vi "Test_WriteValue_InvalidType_Error.vi"(8 "error in (no error)":errorcluster, 11 "TestFormattedStringBinding In":refnum<class "TestFormattedStringBinding.lvclass">) -> (0 "error out":errorcluster, 3 "TestFormattedStringBinding Out":refnum<class "TestFormattedStringBinding.lvclass">)   [LabVIEW 2017, in "TestFormattedStringBinding.lvclass"]
uses:
  TestFormattedStringBinding.lvclass
  Source/Concrete/FormattedStringBinding/FormattedStringBinding.lvclass/FormattedStringBinding.ctl
  Source/Concrete/FormattedStringBinding/FormattedStringBinding.lvclass
  C:/Git/composed-transport/Source/Concrete/TerminalValueBinding/TerminalValueBinding.lvclass
  C:/Git/composed-transport/Source/ITransport/ITransport.lvclass
  <vilib>/Utility/error.llb/Error Cluster From Error Code.vi
  Source/Concrete/TerminalValueBinding/Construct Terminal Value Binding.vi
  Source/ITransport/ITransport.lvclass
panel:
  in  "String":string
  out "Return Error":errorcluster
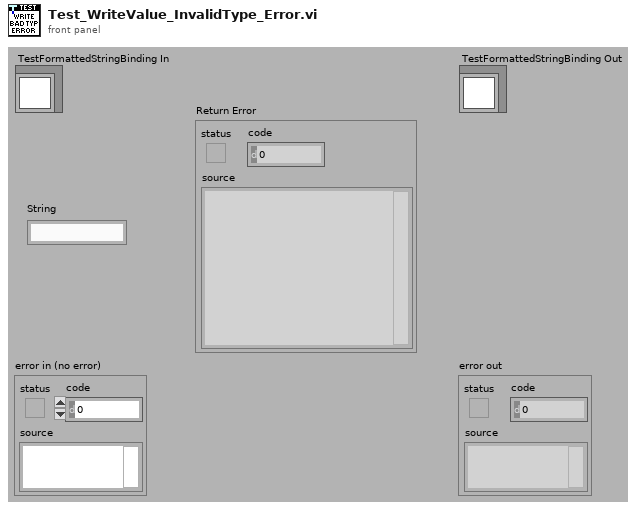
[diagram p1: front panel]
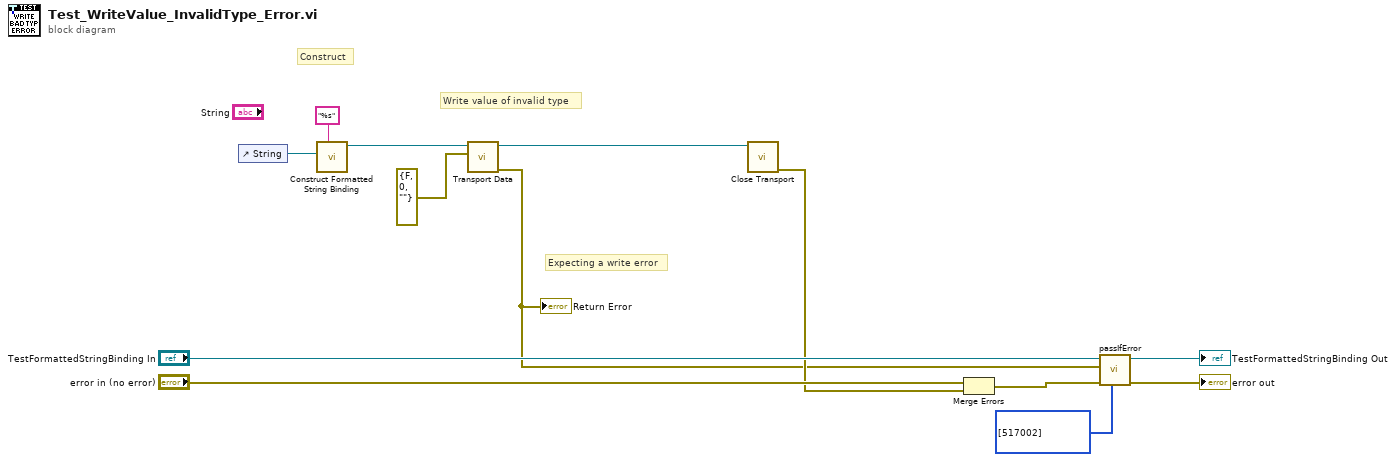
[diagram p0: block diagram]
diagram:
  # "Expecting a write error"
  # "Construct"
  # "Write value of invalid type"
  n1 = control-ref of="String"() -> (w1:refnum<vi>)
  n2 = call "Construct Formatted String Binding.vi"("Format String"="%s", "Str Refnum"=w1) -> ("FormattedStringBinding"=w9:refnum<class "FormattedStringBinding.lvclass">)  [unwired: 8 in, 1 out]
  n3 = call "Transport Data.vi"("Value"=errorcluster {"status"=FALSE, "code"=0, "source"=""} ("error constant"), "ITransport in"=w9) -> ("error out"=w4:errorcluster, "ITransport out"=w7:refnum<class "FormattedStringBinding.lvclass">)  [unwired: 8 in]
  "Return Error" <- w4
  n4 = call-dynamic "Close Transport.vi"("ITransport in"=w7) -> ("error out"=w6:errorcluster)  [unwired: 10 in]
  n5 = Merge Errors("error in (no error)", w6) -> (w8:errorcluster)
  n6 = call-dynamic "passIfError.vi"("passing error codes (default = any error code)"=i32[] [517002], "error in (no error)"=w8, "error"=w4, "TestCase in"="TestFormattedStringBinding In") -> ("error out"=→"error out":errorcluster, "TestCase out"=→"TestFormattedStringBinding Out":refnum<class "TestFormattedStringBinding.lvclass">)  [unwired: 6 in]
